vi "cd_io.vi"(1 "INPUT":cluster{"c2":bool, "c1":bool, "c0":bool}) -> (0 "OUTPUT":T1)   [LabVIEW 2013]
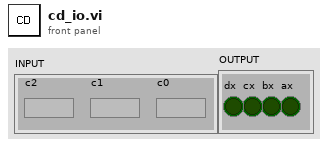
[diagram p1: front panel]
types:
  T1 = cluster{"ax":bool, "bx":bool, "cx":bool, "dx":bool}
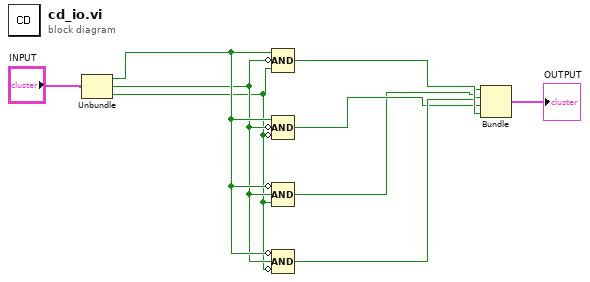
[diagram p0: block diagram]
diagram:
  n1 = Unbundle("INPUT") -> ("c2"=w8:bool, "c1"=w7:bool, "c0"=w6:bool)
  n2 = Compound Arithmetic op=AND(w8, invert w7, w6) -> (w4:bool)
  n3 = Compound Arithmetic op=AND(w8, invert w7, invert w6) -> (w2:bool)
  n4 = Compound Arithmetic op=AND(invert w8, w7, w6) -> (w1:bool)
  n5 = Compound Arithmetic op=AND(invert w8, w7, invert w6) -> (w3:bool)
  n6 = Bundle(w3, w1, w2, w4) -> (→"OUTPUT":cluster{bool, bool, bool, bool})  [unwired: 1 in]
